vi "Write Cycle.vi"(8 "error in (no error)":errorcluster, 10 "Cycle":bool, 11 "Change Speaker Switch State in":refnum<class "Change Speaker Switch State.lvclass">) -> (0 "error out":errorcluster, 3 "Change Speaker Switch State out":refnum<class "Change Speaker Switch State.lvclass">)   [LabVIEW 2014, in "ePAS Library.lvlib" / "Change Speaker Switch State.lvclass"]
uses:
  Change Speaker Switch State.lvclass
  Change Speaker Switch State.lvclass/Change Speaker Switch State.ctl
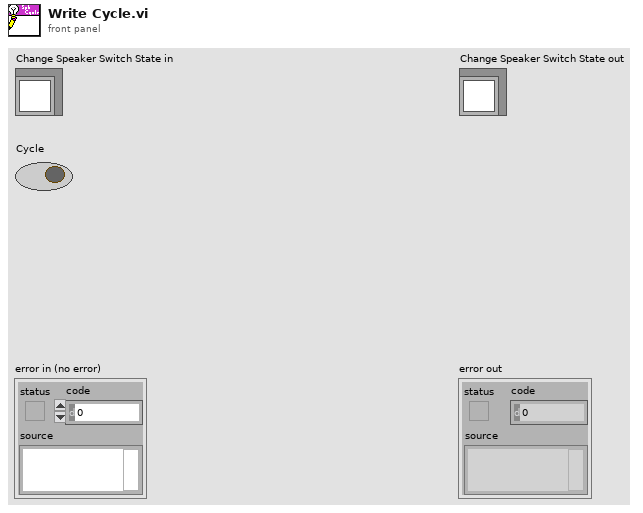
[diagram p1: front panel]
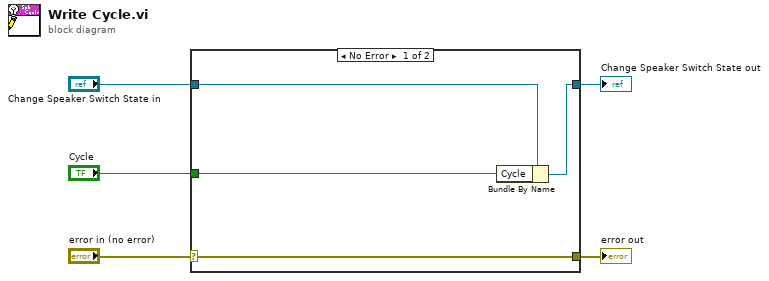
[diagram p0: block diagram]
diagram:
  n1 = case shown="No Error" "error in (no error)" {
    selector: "error in (no error)" -> [w9 w10]
    tunnel: [w9 w10] -> w4
    tunnel: [w7 w11] -> w2
    tunnel: "Change Speaker Switch State in" -> [w8 w11]
    tunnel: "Cycle" -> [w6 _]
    frame No Error {
      n2 = Bundle By Name(cluster=w8, "Cycle"=w6) -> (w7:refnum<class "Change Speaker Switch State.lvclass">)
    }
    frame Error {
    }
  }
  "error out" <- w4
  "Change Speaker Switch State out" <- w2
